vi "global IOC database.vi"() -> ()   [LabVIEW 2023]
uses:
  control/epics database.ctl
panel:
  out "Epics Database":T1[](array[typedef])=[{"IOC"="hama_l9421_02_1", "db"="hama_l9421_02", "Field Values"=["record", "ca", "prefix", "label", "type"], "Values"=[["bo", "$(XSOURCE):checkhardware", "VAL", "checkhardware", "SET"], ["stringin", "$(XSOURCE):model", "VAL", "status", "GET"], ["bo", "$(XSOURCE):reset", "VAL", "reset", "SET"], ["ao", "$(XSOURCE):setcurrent", "VAL", "setcurrent", "SET"], ["ao", "$(XSOURCE):setvoltage", "VAL", "setvoltage", "SET"], ["ai", "$(XSOURCE):sh_battery", "VAL", "show_battery", "GET"], ["ai", "$(XSOURCE):sh_cu", "VAL", "current", "GET"], ["ai", "$(XSOURCE):sh_hv", "VAL", "tension", "GET"], ["bo", "$(XSOURCE):showwarmup", "VAL", "showwarmup", "SET"], ["ai", "$(XSOURCE):sh_pattern_a", "VAL", "warmup_a", "GET"], ["ai", "$(XSOURCE):sh_pattern_b", "VAL", "warmup_b", "GET"], ["ai", "$(XSOURCE):sh_preheating", "VAL", "show_preheating", "GET"], ["ai", "$(XSOURCE):sh_warmup", "VAL", "ahowwarmup", "GET"], ["bo", "$(XSOURCE):startingwarmup", "VAL", "reqwarmup", "SET"], ["ai", "$(XSOURCE):sh_status", "VAL", "showstatus", "GET"], ["ai", "$(XSOURCE):gethardware", "VAL", "showhardware", "GET"], ["bo", "$(XSOURCE):switch_onoff", "VAL", "switch_hv", "SET"]], "Type"="sources", "Card"=1, "Num Dev"=1}, {"IOC"="mm4006_1", "db"="motor ca", "Field Values"=["record", "ca", "prefix", "label", "type"], "Values"=[["stringin", "$(MOT):model", "VAL", "status", "GET"], ["bo", "$(MOT):reqstatus_$(card)_$(axis)", "VAL", "reqstatus", "SET"], ["stringin", "$(MOT):status_$(card)_$(axis)", "VAL", "getstatus", "GET"], ["bo", "$(MOT):reqmotor_$(card)_$(axis)", "VAL", "reqmotor", "SET"], ["stringin", "$(MOT):moving_$(card)_$(axis)", "VAL", "getmoving", "GET"], ["bo", "$(MOT):reqinit_$(card)_$(axis)", "VAL", "reqinit", "SET"], ["bo", "$(MOT):reqhome_$(card)_$(axis)", "VAL", "reqhome", "SET"], ["bo", "$(MOT):reqpos_$(card)_$(axis)", "VAL", "reqpos", "SET"], ["ai", "$(MOT):pos_$(card)_$(axis)", "VAL", "pos", "GET"], ["ao", "$(MOT):setma_$(card)_$(axis)", "VAL", "moveabs", "SET"], ["ao", "$(MOT):setmr_$(card)_$(axis)", "VAL", "moverel", "SET"], ["stringin", "$(MOT):err_$(card)_$(axis)", "VAL", "error", "GET"], ["bo", "$(MOT):reqmoving_$(card)_$(axis)", "VAL", "reqmoving", "SET"]], "Type"="motors", "Card"=1, "Num Dev"=4}, {"IOC"="pi_1", "db"="motor ca", "Field Values"=["record", "ca", "prefix", "label", "type"], "Values"=[["stringin", "$(MOT):model", "VAL", "status", "GET"], ["bo", "$(MOT):reqstatus_$(card)_$(axis)", "VAL", "reqstatus", "SET"], ["stringin", "$(MOT):status_$(card)_$(axis)", "VAL", "getstatus", "GET"], ["bo", "$(MOT):reqmotor_$(card)_$(axis)", "VAL", "reqmotor", "SET"], ["stringin", "$(MOT):moving_$(card)_$(axis)", "VAL", "getmoving", "GET"], ["bo", "$(MOT):reqinit_$(card)_$(axis)", "VAL", "reqinit", "SET"], ["bo", "$(MOT):reqhome_$(card)_$(axis)", "VAL", "reqhome", "SET"], ["bo", "$(MOT):reqpos_$(card)_$(axis)", "VAL", "reqpos", "SET"], ["ai", "$(MOT):pos_$(card)_$(axis)", "VAL", "pos", "GET"], ["ao", "$(MOT):setma_$(card)_$(axis)", "VAL", "moveabs", "SET"], ["ao", "$(MOT):setmr_$(card)_$(axis)", "VAL", "moverel", "SET"], ["stringin", "$(MOT):err_$(card)_$(axis)", "VAL", "error", "GET"], ["bo", "$(MOT):reqmoving_$(card)_$(axis)", "VAL", "reqmoving", "SET"]], "Type"="motors", "Card"=3, "Num Dev"=1}, {"IOC"="pi_2", "db"="motor ca", "Field Values"=["record", "ca", "prefix", "label", "type"], "Values"=[["stringin", "$(MOT):model", "VAL", "status", "GET"], ["bo", "$(MOT):reqstatus_$(card)_$(axis)", "VAL", "reqstatus", "SET"], ["stringin", "$(MOT):status_$(card)_$(axis)", "VAL", "getstatus", "GET"], ["bo", "$(MOT):reqmotor_$(card)_$(axis)", "VAL", "reqmotor", "SET"], ["stringin", "$(MOT):moving_$(card)_$(axis)", "VAL", "getmoving", "GET"], ["bo", "$(MOT):reqinit_$(card)_$(axis)", "VAL", "reqinit", "SET"], ["bo", "$(MOT):reqhome_$(card)_$(axis)", "VAL", "reqhome", "SET"], ["bo", "$(MOT):reqpos_$(card)_$(axis)", "VAL", "reqpos", "SET"], ["ai", "$(MOT):pos_$(card)_$(axis)", "VAL", "pos", "GET"], ["ao", "$(MOT):setma_$(card)_$(axis)", "VAL", "moveabs", "SET"], ["ao", "$(MOT):setmr_$(card)_$(axis)", "VAL", "moverel", "SET"], ["stringin", "$(MOT):err_$(card)_$(axis)", "VAL", "error", "GET"], ["bo", "$(MOT):reqmoving_$(card)_$(axis)", "VAL", "reqmoving", "SET"]], "Type"="motors", "Card"=1, "Num Dev"=1}, {"IOC"="ortec_1", "db"="ort_994", "Field Values"=["record", "ca", "prefix", "label", "type"], "Values"=[["stringin", "$(DETECT):model", "VAL", "status", "GET"], ["stringin", "$(DETECT):init", "VAL", "reqinit", "SET"], ["stringout", "$(DETECT):setdisplay", "VAL", "setdisplay", "SET"], ["stringout", "$(DETECT):setcoupr", "VAL", "settime", "SET"], ["stringin", "$(DETECT):getcoupr", "VAL", "gettime", "GET"], ["bo", "$(DETECT):readcount", "VAL", "reqdata", "SET"], ["calc", "$(DETECT):count", "VAL", "data", "GET"], ["stringin", "$(DETECT):clearcount", "VAL", "reset", "SET"], ["bo", "$(DETECT):showdisplay", "VAL", "reqdisplay", "SET"], ["bi", "$(DETECT):getDisplay", "VAL", "display", "GET"], ["bo", "$(DETECT):starting", "VAL", "reqacq", "SET"]], "Type"="detectors", "Card"=1, "Num Dev"=1}, {"IOC"="cts_rt_fpga", "db"="cts_rt_fpga", "Field Values"=["record", "ca", "prefix", "label", "type"], "Values"=[["bi", "$(RT_FPGA):status", "VAL", "status", "GET"], ["bi", "$(RT_FPGA):hv_on", "VAL", "hv", "GET"], ["bi", "$(RT_FPGA):closed_door", "VAL", "door", "GET"], ["bi", "$(RT_FPGA):closed_extra_door", "VAL", "exdoor", "GET"], ["bi", "$(RT_FPGA):shutter_opened", "VAL", "shutter", "GET"], ["bo", "$(RT_FPGA):high_energies", "VAL", "reqhe", "SET"], ["bo", "$(RT_FPGA):power_supply", "VAL", "reqps", "SET"], ["bo", "$(RT_FPGA):shutter", "VAL", "reqshutter", "SET"]], "Type"="rt_fpga", "Card"=1, "Num Dev"=1}]
  in  "Value IOC":string[][](array[string])=[["hama_l9421_02_1", "192.168.149.102", "sources", "hama_l9421_02", "20003", "ham_l9421_02_1"], ["mm4006_1", "192.168.149.102", "motors", "motor ca", "20001", "mm4006IOC"], ["pi_1", "192.168.149.102", "motors", "motor ca", "20004", "piIOC"], ["pi_2", "192.168.149.102", "motors", "motor ca", "20005", "piIOC2"], ["ortec_1", "192.168.149.102", "detectors", "ort_994", "20002", "ort_994"], ["cts_rt_fpga", "192.168.149.110", "rt_fpga", "cts_rt_fpga", "NULL", "cts_rt_fpga"]]
  in  "Field Name IOC":string[](array[string])=["ioc", "server", "type", "db", "port", "family"]
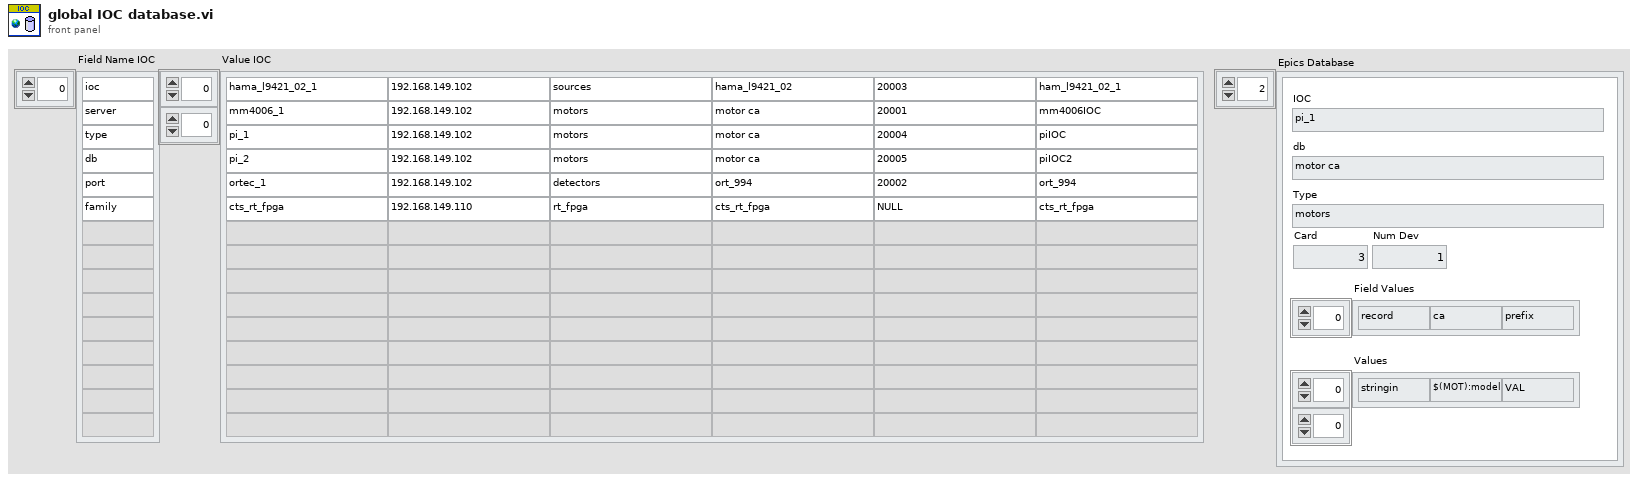
[diagram p1: front panel]
types:
  T1 = typedef "epics database.ctl" = cluster{"IOC":string, "db":string, "Field Values":string[], "Values":string[][], "Type":string, "Card":u16, "Num Dev":u16}
diagram:
